vi "CRC校验.vi"(1 "字符串":string) -> (0 "十六进制整型字符串":string)   [LabVIEW 2012]
panel:
  # "01 03 0400 0004"
  # "4539"
  # "010304000004"
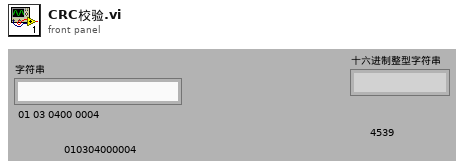
[diagram p1: front panel]
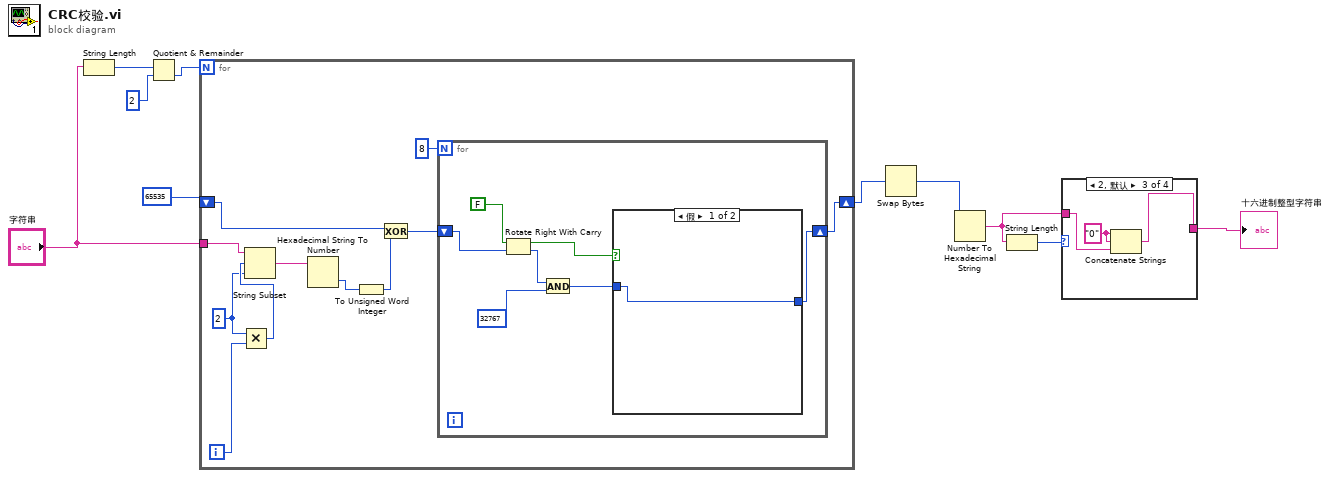
[diagram p0: block diagram]
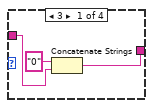
[diagram p2: hidden frame]
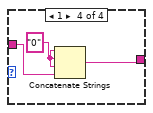
[diagram p4: hidden frame]
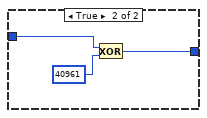
[diagram p5: hidden frame]
diagram:
  n1 = String Length(string="字符串") -> (length=w10:i32)
  n2 = Quotient & Remainder(x=w10, y=2) -> (floor(x/y)=w4:i32)  [unwired: 1 out]
  n3 = for {
    N: w4 -> [_]
    shift-right: [w12] -> w9
    shift-left: u16 65535 -> [w16]
    tunnel: "字符串" -> [w11]
    i -> [w20]
    w18 = 2
    n4 = Multiply(x=w18, y=w20) -> (x*y=w19:i32)
    n5 = String Subset(string=w11, offset (0)=w19, length (rest)=w18) -> (substring=w21:string)
    n6 = Hexadecimal String To Number(string=w21) -> (number=w17:u32)  [unwired: 2 in, 1 out]
    n7 = To Unsigned Word Integer(number=w17) -> (unsigned 16bit integer=w15:u16)
    n8 = Exclusive Or(1:w15, 2:w16) -> (0:w14:u16)
    n9 = for {
      N: 8 -> [_]
      shift-right: [w23] -> w12
      shift-left: w14 -> [w28]
      n10 = Rotate Right With Carry(2:w28, 3:FALSE) -> (0:w26:u16, 1:w22:bool)
      n11 = And(x=w26, y=u16 32767) -> (x .and. y?=w24:u16)
      n12 = case shown="假" w22 {
        tunnel: w24 -> [w29 w31]
        tunnel: [w29 w30] -> w23
        frame False {
        }
        frame True {
          n13 = Exclusive Or(1:u16 40961, 2:w31) -> (0:w30:u16)
        }
      }
    }
  }
  n14 = Swap Bytes(anything=w9) -> (byte swapped=w7:u16)
  n15 = Number To Hexadecimal String(2:w7) -> (0:w2:string)  [unwired: 1 in]
  n16 = String Length(string=w2) -> (length=w3:i32)
  n17 = case shown="2, 默认" w3 {
    tunnel: w2 -> [w34 w36 w38 w42]
    tunnel: [w33 w36 w37 w40] -> w1
    frame 3 {
      n18 = Concatenate Strings("0" ("字符串"), w34) -> (w33:string)
    }
    frame 4 {
    }
    frame 2, Default {
      w39 = "0" ("字符串")
      n19 = Concatenate Strings(w39, w39, w38) -> (w37:string)
    }
    frame 1 {
      w41 = "0" ("字符串")
      n20 = Concatenate Strings(w41, w41, w41, w42) -> (w40:string)
    }
  }
  "十六进制整型字符串" <- w1
